vi "Remove non-unique Strings.vi"(11 "String Array in":cluster{"Path Identifiers":string[]}[](array[cluster])) -> (2 "Removed Strings":string[](array[string]), 3 "String Array out":cluster{"Array":string[]}[](array[cluster]))   [LabVIEW 2019, in "Project.Dependencies Finder.lvlib"]
doc: "Remove all strings that are non unique in the given sets of strings."
uses:
  Project.Dependencies Finder.lvlib
  e42de9b8-5810-47d0-a18d-f660b697bb01.vi
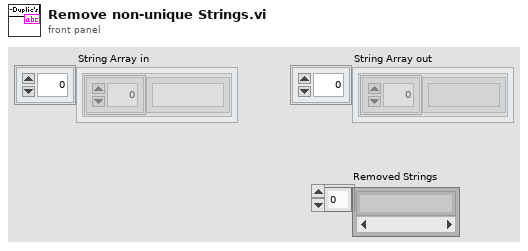
[diagram p1: front panel]
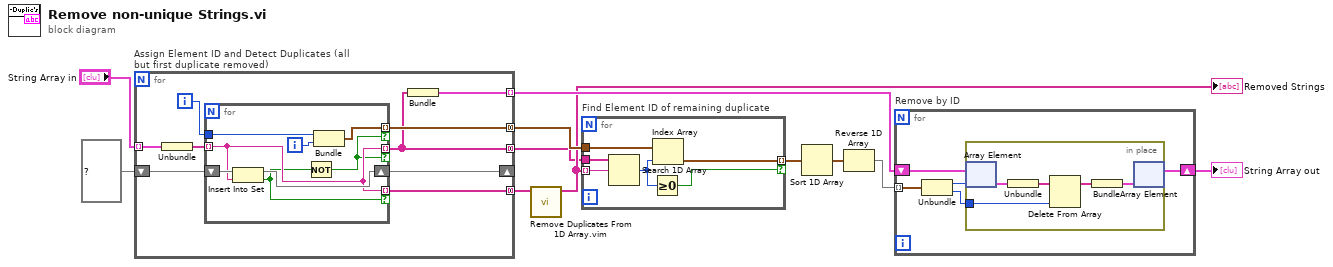
[diagram p0: block diagram]
diagram:
  n1 = for "Assign Element ID and Detect Duplicates (all but first duplicate removed)" {
    shift-right: [w16] -> _
    shift-left: set{string} {} ("set") -> [w19]
    tunnel: [w12] -> w8 mode=indexing
    tunnel: [w18] -> w5 mode=concatenating
    tunnel: [w17] -> w2 mode=concatenating
    tunnel: [w13] -> w3 mode=concatenating
    tunnel: "String Array in" -> [w15] mode=indexing
    i -> [w20]
    n2 = Unbundle(w15) -> ("Path Identifiers"=w14:string[])
    n3 = for {
      tunnel: w14 -> [w23] mode=indexing
      tunnel: [w23] -> w13 mode=indexing if=w21
      tunnel: w20 -> [w27]
      tunnel: [w26] -> w18 mode=indexing if=w21
      shift-right: [w24] -> w16
      shift-left: w19 -> [w25]
      tunnel: [w23] -> w17 mode=indexing if=w22
      i -> [w28]
      n4 = Insert Into Set(10:w23, 11:w25) -> (2:w22:bool, 3:w24:set{string})
      n5 = Not(x=w22) -> (.not. x?=w21:bool)
      n6 = Bundle(w27, w28) -> (w26:cluster{i32, i32})  [unwired: 1 in]
    }
    n7 = Bundle(w13) -> (w12:cluster{string[]})  [unwired: 1 in]
  }
  n8 = call "Remove Duplicates From 1D Array.vim"("array"=w2) -> ("array with duplicates removed"=w4:string[])  [unwired: 10 in]
  "Removed Strings" <- w4
  n9 = for "Find Element ID of remaining duplicate" {
    tunnel: w3 -> [w34]
    tunnel: w4 -> [w33] mode=indexing
    tunnel: w5 -> [w32]
    tunnel: [w30] -> w6 mode=indexing if=w29
    n10 = Search 1D Array(1D array=w34, element=w33) -> (index of element=w31:i32)  [unwired: 1 in]
    n11 = Greater Or Equal To 0?(x=w31) -> (x >= 0?=w29:bool)
    n12 = Index Array(array=w32, index=w31) -> (element=w30:cluster{i32, i32})
  }
  n13 = Sort 1D Array(array=w6) -> (sorted array=w7:cluster{i32, i32}[])
  n14 = Reverse 1D Array(array=w7) -> (reversed array=w9:cluster{i32, i32}[])
  n15 = for "Remove by ID" {
    shift-right: [w35] -> w11
    shift-left: w8 -> [w38]
    tunnel: w9 -> [w39] mode=indexing
    n16 = Unbundle(w39) -> (w37:i32, w36:i32)
    n17 = in-place {
      in-place-border: w36 -> [w44]
      n18 = in-place-array #1(w38, w37) -> (w43:cluster{string[]})
      n19 = Unbundle(w43) -> (w42:string[])
      n20 = Delete From Array(array=w42, index=w44) -> (array with subset deleted=w41:string[])  [unwired: 1 in, 1 out]
      n21 = Bundle(w41) -> (w40:cluster{string[]})  [unwired: 1 in]
      n22 = in-place-array #1(w40) -> (w35:cluster{string[]}[])  [unwired: 1 out]
    }
  }
  "String Array out" <- w11
